vi "Scoreboard.vi"(3 "B득점":u32, 11 "A득점":u32) -> ()   [LabVIEW 2020]
panel:
  out "7SegmentB1":T1
  out "7SegmentB10":T1
  out "7SegmentB100":T1
  out "7SegmentA1":T1
  out "7SegmentA10":T1
  out "7SegmentA100":T1
  # "A득점"
  # "B득점"
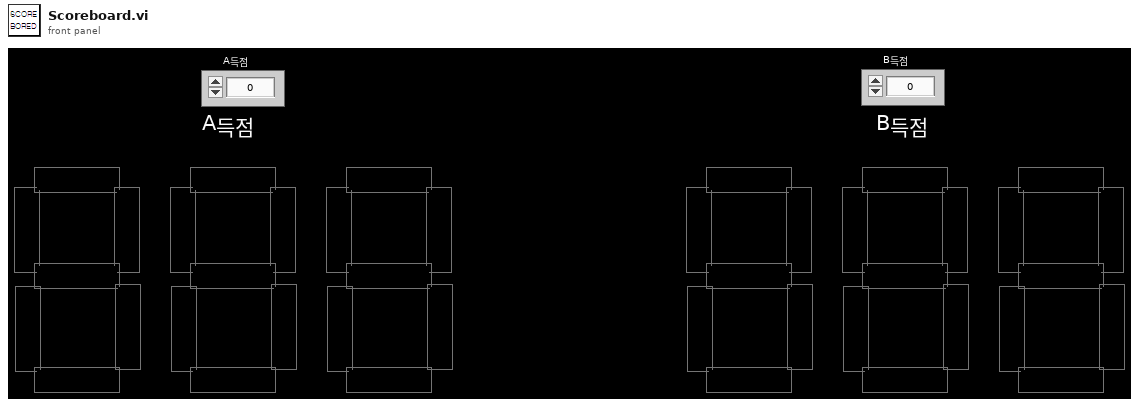
[diagram p1: front panel]
types:
  T1 = cluster{"Led 4":bool, "Led":bool, "Led 3":bool, "Led 2":bool, "Led 5":bool, "Led 6":bool, "Led 7":bool}
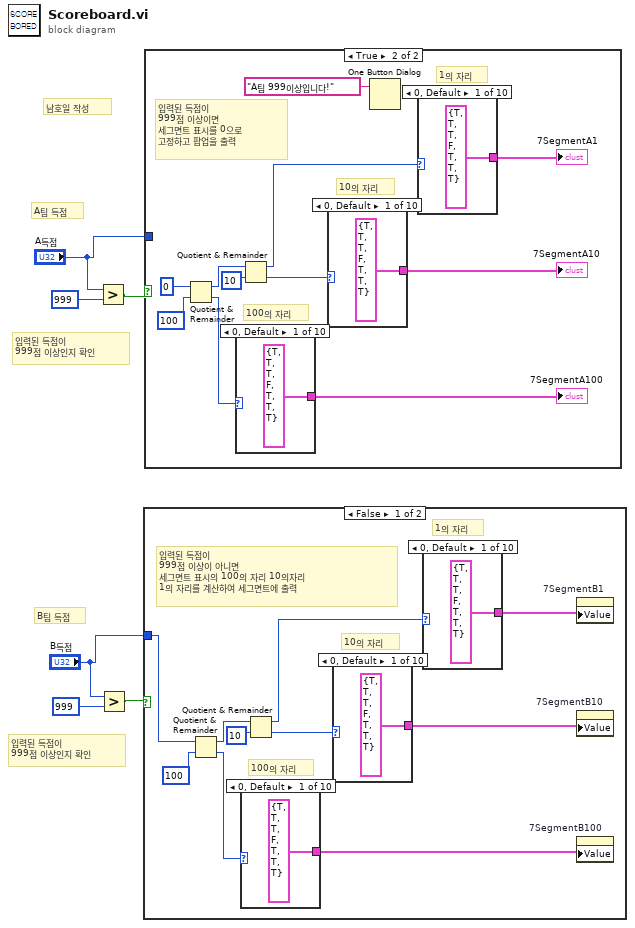
[diagram p0: block diagram]
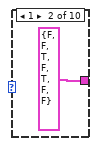
[diagram p2: hidden frame]
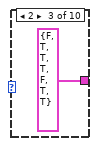
[diagram p3: hidden frame]
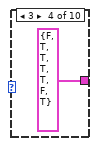
[diagram p4: hidden frame]
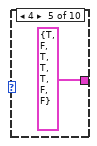
[diagram p5: hidden frame]
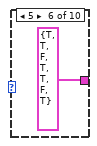
[diagram p6: hidden frame]
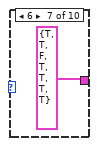
[diagram p7: hidden frame]
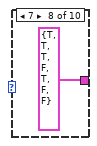
[diagram p8: hidden frame]
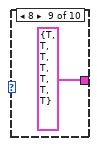
[diagram p9: hidden frame]
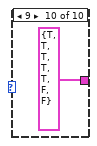
[diagram p10: hidden frame]
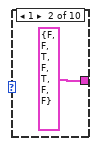
[diagram p11: hidden frame]
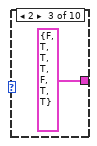
[diagram p12: hidden frame]
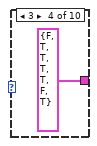
[diagram p13: hidden frame]
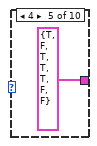
[diagram p14: hidden frame]
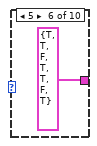
[diagram p15: hidden frame]
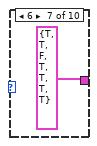
[diagram p16: hidden frame]
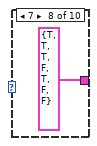
[diagram p17: hidden frame]
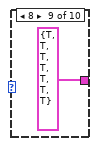
[diagram p18: hidden frame]
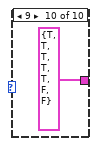
[diagram p19: hidden frame]
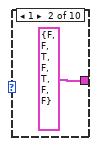
[diagram p20: hidden frame]
diagram:
  # "입력된 득점이 \n999점 이상인지 확인"
  # "입력된 득점이 \n999점 이상인지 확인"
  # "남호일 작성"
  # "B팀 득점"
  # "A팀 득점"
  n1 = Greater?(x="A득점", y=u32 999) -> (0:w2:bool)
  n2 = Greater?(x="B득점", y=u32 999) -> (0:w1:bool)
  n3 = case shown="False" w1 {
    tunnel: "B득점" -> [w7 _]
    frame False {
      # "입력된 득점이 \n999점 이상이 아니면 \n세그면트 표시의 100의 자리 10의자리 \n1의 자리를 계산하여 세그면트에 출력"
      # "1의 자리"
      # "10의 자리"
      # "100의 자리"
      n4 = Quotient & Remainder(x=w7, y=u32 100) -> (x-y*floor(x/y)=w15:u32, floor(x/y)=w14:u32)
      n5 = case shown="0, Default" w14 {
        tunnel: [T1 {"Led 4"=TRUE, "Led"=TRUE, "Led 3"=TRUE, "Led 2"=FALSE, "Led 5"=TRUE, "Led 6"=TRUE, "Led 7"=TRUE} ("7Segment10min") T1 {"Led 4"=FALSE, "Led"=FALSE, "Led 3"=TRUE, "Led 2"=FALSE, "Led 5"=TRUE, "Led 6"=FALSE, "Led 7"=FALSE} ("7Segment10min") T1 {"Led 4"=FALSE, "Led"=TRUE, "Led 3"=TRUE, "Led 2"=TRUE, "Led 5"=FALSE, "Led 6"=TRUE, "Led 7"=TRUE} ("7Segment10min") T1 {"Led 4"=FALSE, "Led"=TRUE, "Led 3"=TRUE, "Led 2"=TRUE, "Led 5"=TRUE, "Led 6"=FALSE, "Led 7"=TRUE} ("7Segment10min") T1 {"Led 4"=TRUE, "Led"=FALSE, "Led 3"=TRUE, "Led 2"=TRUE, "Led 5"=TRUE, "Led 6"=FALSE, "Led 7"=FALSE} ("7Segment10min") T1 {"Led 4"=TRUE, "Led"=TRUE, "Led 3"=FALSE, "Led 2"=TRUE, "Led 5"=TRUE, "Led 6"=FALSE, "Led 7"=TRUE} ("7Segment10min") T1 {"Led 4"=TRUE, "Led"=TRUE, "Led 3"=FALSE, "Led 2"=TRUE, "Led 5"=TRUE, "Led 6"=TRUE, "Led 7"=TRUE} ("7Segment10min") T1 {"Led 4"=TRUE, "Led"=TRUE, "Led 3"=TRUE, "Led 2"=FALSE, "Led 5"=TRUE, "Led 6"=FALSE, "Led 7"=FALSE} ("7Segment10min") T1 {"Led 4"=TRUE, "Led"=TRUE, "Led 3"=TRUE, "Led 2"=TRUE, "Led 5"=TRUE, "Led 6"=TRUE, "Led 7"=TRUE} ("7Segment10min") T1 {"Led 4"=TRUE, "Led"=TRUE, "Led 3"=TRUE, "Led 2"=TRUE, "Led 5"=TRUE, "Led 6"=FALSE, "Led 7"=FALSE} ("7Segment10min")] -> w10
        frame 0, Default {
        }
        frame 1 {
        }
        frame 2 {
        }
        frame 3 {
        }
        frame 4 {
        }
        frame 5 {
        }
        frame 6 {
        }
        frame 7 {
        }
        frame 8 {
        }
        frame 9 {
        }
      }
      n6 = Quotient & Remainder(x=w15, y=u32 10) -> (x-y*floor(x/y)=w11:u32, floor(x/y)=w12:u32)
      n7 = case shown="0, Default" w12 {
        tunnel: [T1 {"Led 4"=TRUE, "Led"=TRUE, "Led 3"=TRUE, "Led 2"=FALSE, "Led 5"=TRUE, "Led 6"=TRUE, "Led 7"=TRUE} ("7Segment10min") T1 {"Led 4"=FALSE, "Led"=FALSE, "Led 3"=TRUE, "Led 2"=FALSE, "Led 5"=TRUE, "Led 6"=FALSE, "Led 7"=FALSE} ("7Segment10min") T1 {"Led 4"=FALSE, "Led"=TRUE, "Led 3"=TRUE, "Led 2"=TRUE, "Led 5"=FALSE, "Led 6"=TRUE, "Led 7"=TRUE} ("7Segment10min") T1 {"Led 4"=FALSE, "Led"=TRUE, "Led 3"=TRUE, "Led 2"=TRUE, "Led 5"=TRUE, "Led 6"=FALSE, "Led 7"=TRUE} ("7Segment10min") T1 {"Led 4"=TRUE, "Led"=FALSE, "Led 3"=TRUE, "Led 2"=TRUE, "Led 5"=TRUE, "Led 6"=FALSE, "Led 7"=FALSE} ("7Segment10min") T1 {"Led 4"=TRUE, "Led"=TRUE, "Led 3"=FALSE, "Led 2"=TRUE, "Led 5"=TRUE, "Led 6"=FALSE, "Led 7"=TRUE} ("7Segment10min") T1 {"Led 4"=TRUE, "Led"=TRUE, "Led 3"=FALSE, "Led 2"=TRUE, "Led 5"=TRUE, "Led 6"=TRUE, "Led 7"=TRUE} ("7Segment10min") T1 {"Led 4"=TRUE, "Led"=TRUE, "Led 3"=TRUE, "Led 2"=FALSE, "Led 5"=TRUE, "Led 6"=FALSE, "Led 7"=FALSE} ("7Segment10min") T1 {"Led 4"=TRUE, "Led"=TRUE, "Led 3"=TRUE, "Led 2"=TRUE, "Led 5"=TRUE, "Led 6"=TRUE, "Led 7"=TRUE} ("7Segment10min") T1 {"Led 4"=TRUE, "Led"=TRUE, "Led 3"=TRUE, "Led 2"=TRUE, "Led 5"=TRUE, "Led 6"=FALSE, "Led 7"=FALSE} ("7Segment10min")] -> w9
        frame 0, Default {
        }
        frame 1 {
        }
        frame 2 {
        }
        frame 3 {
        }
        frame 4 {
        }
        frame 5 {
        }
        frame 6 {
        }
        frame 7 {
        }
        frame 8 {
        }
        frame 9 {
        }
      }
      n8 = case shown="0, Default" w11 {
        tunnel: [T1 {"Led 4"=TRUE, "Led"=TRUE, "Led 3"=TRUE, "Led 2"=FALSE, "Led 5"=TRUE, "Led 6"=TRUE, "Led 7"=TRUE} ("7Segment10min") T1 {"Led 4"=FALSE, "Led"=FALSE, "Led 3"=TRUE, "Led 2"=FALSE, "Led 5"=TRUE, "Led 6"=FALSE, "Led 7"=FALSE} ("7Segment10min") T1 {"Led 4"=FALSE, "Led"=TRUE, "Led 3"=TRUE, "Led 2"=TRUE, "Led 5"=FALSE, "Led 6"=TRUE, "Led 7"=TRUE} ("7Segment10min") T1 {"Led 4"=FALSE, "Led"=TRUE, "Led 3"=TRUE, "Led 2"=TRUE, "Led 5"=TRUE, "Led 6"=FALSE, "Led 7"=TRUE} ("7Segment10min") T1 {"Led 4"=TRUE, "Led"=FALSE, "Led 3"=TRUE, "Led 2"=TRUE, "Led 5"=TRUE, "Led 6"=FALSE, "Led 7"=FALSE} ("7Segment10min") T1 {"Led 4"=TRUE, "Led"=TRUE, "Led 3"=FALSE, "Led 2"=TRUE, "Led 5"=TRUE, "Led 6"=FALSE, "Led 7"=TRUE} ("7Segment10min") T1 {"Led 4"=TRUE, "Led"=TRUE, "Led 3"=FALSE, "Led 2"=TRUE, "Led 5"=TRUE, "Led 6"=TRUE, "Led 7"=TRUE} ("7Segment10min") T1 {"Led 4"=TRUE, "Led"=TRUE, "Led 3"=TRUE, "Led 2"=FALSE, "Led 5"=TRUE, "Led 6"=FALSE, "Led 7"=FALSE} ("7Segment10min") T1 {"Led 4"=TRUE, "Led"=TRUE, "Led 3"=TRUE, "Led 2"=TRUE, "Led 5"=TRUE, "Led 6"=TRUE, "Led 7"=TRUE} ("7Segment10min") T1 {"Led 4"=TRUE, "Led"=TRUE, "Led 3"=TRUE, "Led 2"=TRUE, "Led 5"=TRUE, "Led 6"=FALSE, "Led 7"=FALSE} ("7Segment10min")] -> w8
        frame 0, Default {
        }
        frame 1 {
        }
        frame 2 {
        }
        frame 3 {
        }
        frame 4 {
        }
        frame 5 {
        }
        frame 6 {
        }
        frame 7 {
        }
        frame 8 {
        }
        frame 9 {
        }
      }
      n9 = property on="7SegmentB1" class="Clust (strict)"("Value"=w8) -> ()  [unwired: 2 in, 2 out]
      n10 = property on="7SegmentB10" class="Clust (strict)"("Value"=w9) -> ()  [unwired: 2 in, 2 out]
      n11 = property on="7SegmentB100" class="Clust (strict)"("Value"=w10) -> ()  [unwired: 2 in, 2 out]
    }
    frame True {
      # "입력된 득점이 \n999점 이상이면 \n세그면트 표시를 0으로 고정하고 팝업을 출력"
      # "1의 자리"
      # "10의 자리"
      # "100의 자리"
      n12 = Quotient & Remainder(x=u32 0, y=u32 100) -> (x-y*floor(x/y)=w56:u32, floor(x/y)=w55:u32)
      n13 = case shown="0, Default" w55 {
        tunnel: [T1 {"Led 4"=TRUE, "Led"=TRUE, "Led 3"=TRUE, "Led 2"=FALSE, "Led 5"=TRUE, "Led 6"=TRUE, "Led 7"=TRUE} ("7Segment10min") T1 {"Led 4"=FALSE, "Led"=FALSE, "Led 3"=TRUE, "Led 2"=FALSE, "Led 5"=TRUE, "Led 6"=FALSE, "Led 7"=FALSE} ("7Segment10min") T1 {"Led 4"=FALSE, "Led"=TRUE, "Led 3"=TRUE, "Led 2"=TRUE, "Led 5"=FALSE, "Led 6"=TRUE, "Led 7"=TRUE} ("7Segment10min") T1 {"Led 4"=FALSE, "Led"=TRUE, "Led 3"=TRUE, "Led 2"=TRUE, "Led 5"=TRUE, "Led 6"=FALSE, "Led 7"=TRUE} ("7Segment10min") T1 {"Led 4"=TRUE, "Led"=FALSE, "Led 3"=TRUE, "Led 2"=TRUE, "Led 5"=TRUE, "Led 6"=FALSE, "Led 7"=FALSE} ("7Segment10min") T1 {"Led 4"=TRUE, "Led"=TRUE, "Led 3"=FALSE, "Led 2"=TRUE, "Led 5"=TRUE, "Led 6"=FALSE, "Led 7"=TRUE} ("7Segment10min") T1 {"Led 4"=TRUE, "Led"=TRUE, "Led 3"=FALSE, "Led 2"=TRUE, "Led 5"=TRUE, "Led 6"=TRUE, "Led 7"=TRUE} ("7Segment10min") T1 {"Led 4"=TRUE, "Led"=TRUE, "Led 3"=TRUE, "Led 2"=FALSE, "Led 5"=TRUE, "Led 6"=FALSE, "Led 7"=FALSE} ("7Segment10min") T1 {"Led 4"=TRUE, "Led"=TRUE, "Led 3"=TRUE, "Led 2"=TRUE, "Led 5"=TRUE, "Led 6"=TRUE, "Led 7"=TRUE} ("7Segment10min") T1 {"Led 4"=TRUE, "Led"=TRUE, "Led 3"=TRUE, "Led 2"=TRUE, "Led 5"=TRUE, "Led 6"=FALSE, "Led 7"=FALSE} ("7Segment10min")] -> w51
        frame 0, Default {
        }
        frame 1 {
        }
        frame 2 {
        }
        frame 3 {
        }
        frame 4 {
        }
        frame 5 {
        }
        frame 6 {
        }
        frame 7 {
        }
        frame 8 {
        }
        frame 9 {
        }
      }
      "7SegmentB100" <- w51
      n14 = Quotient & Remainder(x=w56, y=u32 10) -> (x-y*floor(x/y)=w52:u32, floor(x/y)=w53:u32)
      n15 = case shown="0, Default" w53 {
        tunnel: [T1 {"Led 4"=TRUE, "Led"=TRUE, "Led 3"=TRUE, "Led 2"=FALSE, "Led 5"=TRUE, "Led 6"=TRUE, "Led 7"=TRUE} ("7Segment10min") T1 {"Led 4"=FALSE, "Led"=FALSE, "Led 3"=TRUE, "Led 2"=FALSE, "Led 5"=TRUE, "Led 6"=FALSE, "Led 7"=FALSE} ("7Segment10min") T1 {"Led 4"=FALSE, "Led"=TRUE, "Led 3"=TRUE, "Led 2"=TRUE, "Led 5"=FALSE, "Led 6"=TRUE, "Led 7"=TRUE} ("7Segment10min") T1 {"Led 4"=FALSE, "Led"=TRUE, "Led 3"=TRUE, "Led 2"=TRUE, "Led 5"=TRUE, "Led 6"=FALSE, "Led 7"=TRUE} ("7Segment10min") T1 {"Led 4"=TRUE, "Led"=FALSE, "Led 3"=TRUE, "Led 2"=TRUE, "Led 5"=TRUE, "Led 6"=FALSE, "Led 7"=FALSE} ("7Segment10min") T1 {"Led 4"=TRUE, "Led"=TRUE, "Led 3"=FALSE, "Led 2"=TRUE, "Led 5"=TRUE, "Led 6"=FALSE, "Led 7"=TRUE} ("7Segment10min") T1 {"Led 4"=TRUE, "Led"=TRUE, "Led 3"=FALSE, "Led 2"=TRUE, "Led 5"=TRUE, "Led 6"=TRUE, "Led 7"=TRUE} ("7Segment10min") T1 {"Led 4"=TRUE, "Led"=TRUE, "Led 3"=TRUE, "Led 2"=FALSE, "Led 5"=TRUE, "Led 6"=FALSE, "Led 7"=FALSE} ("7Segment10min") T1 {"Led 4"=TRUE, "Led"=TRUE, "Led 3"=TRUE, "Led 2"=TRUE, "Led 5"=TRUE, "Led 6"=TRUE, "Led 7"=TRUE} ("7Segment10min") T1 {"Led 4"=TRUE, "Led"=TRUE, "Led 3"=TRUE, "Led 2"=TRUE, "Led 5"=TRUE, "Led 6"=FALSE, "Led 7"=FALSE} ("7Segment10min")] -> w49
        frame 0, Default {
        }
        frame 1 {
        }
        frame 2 {
        }
        frame 3 {
        }
        frame 4 {
        }
        frame 5 {
        }
        frame 6 {
        }
        frame 7 {
        }
        frame 8 {
        }
        frame 9 {
        }
      }
      "7SegmentB10" <- w49
      n16 = One Button Dialog(message="B팀 999이상입니다!") -> ()  [unwired: 1 in, 1 out]
      n17 = case shown="0, Default" w52 {
        tunnel: [T1 {"Led 4"=TRUE, "Led"=TRUE, "Led 3"=TRUE, "Led 2"=FALSE, "Led 5"=TRUE, "Led 6"=TRUE, "Led 7"=TRUE} ("7Segment10min") T1 {"Led 4"=FALSE, "Led"=FALSE, "Led 3"=TRUE, "Led 2"=FALSE, "Led 5"=TRUE, "Led 6"=FALSE, "Led 7"=FALSE} ("7Segment10min") T1 {"Led 4"=FALSE, "Led"=TRUE, "Led 3"=TRUE, "Led 2"=TRUE, "Led 5"=FALSE, "Led 6"=TRUE, "Led 7"=TRUE} ("7Segment10min") T1 {"Led 4"=FALSE, "Led"=TRUE, "Led 3"=TRUE, "Led 2"=TRUE, "Led 5"=TRUE, "Led 6"=FALSE, "Led 7"=TRUE} ("7Segment10min") T1 {"Led 4"=TRUE, "Led"=FALSE, "Led 3"=TRUE, "Led 2"=TRUE, "Led 5"=TRUE, "Led 6"=FALSE, "Led 7"=FALSE} ("7Segment10min") T1 {"Led 4"=TRUE, "Led"=TRUE, "Led 3"=FALSE, "Led 2"=TRUE, "Led 5"=TRUE, "Led 6"=FALSE, "Led 7"=TRUE} ("7Segment10min") T1 {"Led 4"=TRUE, "Led"=TRUE, "Led 3"=FALSE, "Led 2"=TRUE, "Led 5"=TRUE, "Led 6"=TRUE, "Led 7"=TRUE} ("7Segment10min") T1 {"Led 4"=TRUE, "Led"=TRUE, "Led 3"=TRUE, "Led 2"=FALSE, "Led 5"=TRUE, "Led 6"=FALSE, "Led 7"=FALSE} ("7Segment10min") T1 {"Led 4"=TRUE, "Led"=TRUE, "Led 3"=TRUE, "Led 2"=TRUE, "Led 5"=TRUE, "Led 6"=TRUE, "Led 7"=TRUE} ("7Segment10min") T1 {"Led 4"=TRUE, "Led"=TRUE, "Led 3"=TRUE, "Led 2"=TRUE, "Led 5"=TRUE, "Led 6"=FALSE, "Led 7"=FALSE} ("7Segment10min")] -> w50
        frame 0, Default {
        }
        frame 1 {
        }
        frame 2 {
        }
        frame 3 {
        }
        frame 4 {
        }
        frame 5 {
        }
        frame 6 {
        }
        frame 7 {
        }
        frame 8 {
        }
        frame 9 {
        }
      }
      "7SegmentB1" <- w50
    }
  }
  n18 = case shown="True" w2 {
    tunnel: "A득점" -> [w88 _]
    frame False {
      # "입력된 득점이 \n999점 이상이 아니면 \n세그면트 표시의 100의 자리 10의자리 \n1의 자리를 계산하여 세그면트에 출력"
      # "1의 자리"
      # "10의 자리"
      # "100의 자리"
      n19 = Quotient & Remainder(x=w88, y=u32 100) -> (x-y*floor(x/y)=w97:u32, floor(x/y)=w96:u32)
      n20 = case shown="0, Default" w96 {
        tunnel: [T1 {"Led 4"=TRUE, "Led"=TRUE, "Led 3"=TRUE, "Led 2"=FALSE, "Led 5"=TRUE, "Led 6"=TRUE, "Led 7"=TRUE} ("7Segment10min") T1 {"Led 4"=FALSE, "Led"=FALSE, "Led 3"=TRUE, "Led 2"=FALSE, "Led 5"=TRUE, "Led 6"=FALSE, "Led 7"=FALSE} ("7Segment10min") T1 {"Led 4"=FALSE, "Led"=TRUE, "Led 3"=TRUE, "Led 2"=TRUE, "Led 5"=FALSE, "Led 6"=TRUE, "Led 7"=TRUE} ("7Segment10min") T1 {"Led 4"=FALSE, "Led"=TRUE, "Led 3"=TRUE, "Led 2"=TRUE, "Led 5"=TRUE, "Led 6"=FALSE, "Led 7"=TRUE} ("7Segment10min") T1 {"Led 4"=TRUE, "Led"=FALSE, "Led 3"=TRUE, "Led 2"=TRUE, "Led 5"=TRUE, "Led 6"=FALSE, "Led 7"=FALSE} ("7Segment10min") T1 {"Led 4"=TRUE, "Led"=TRUE, "Led 3"=FALSE, "Led 2"=TRUE, "Led 5"=TRUE, "Led 6"=FALSE, "Led 7"=TRUE} ("7Segment10min") T1 {"Led 4"=TRUE, "Led"=TRUE, "Led 3"=FALSE, "Led 2"=TRUE, "Led 5"=TRUE, "Led 6"=TRUE, "Led 7"=TRUE} ("7Segment10min") T1 {"Led 4"=TRUE, "Led"=TRUE, "Led 3"=TRUE, "Led 2"=FALSE, "Led 5"=TRUE, "Led 6"=FALSE, "Led 7"=FALSE} ("7Segment10min") T1 {"Led 4"=TRUE, "Led"=TRUE, "Led 3"=TRUE, "Led 2"=TRUE, "Led 5"=TRUE, "Led 6"=TRUE, "Led 7"=TRUE} ("7Segment10min") T1 {"Led 4"=TRUE, "Led"=TRUE, "Led 3"=TRUE, "Led 2"=TRUE, "Led 5"=TRUE, "Led 6"=FALSE, "Led 7"=FALSE} ("7Segment10min")] -> w91
        frame 0, Default {
        }
        frame 1 {
        }
        frame 2 {
        }
        frame 3 {
        }
        frame 4 {
        }
        frame 5 {
        }
        frame 6 {
        }
        frame 7 {
        }
        frame 8 {
        }
        frame 9 {
        }
      }
      n21 = Quotient & Remainder(x=w97, y=u32 10) -> (x-y*floor(x/y)=w94:u32, floor(x/y)=w95:u32)
      n22 = case shown="0, Default" w95 {
        tunnel: [T1 {"Led 4"=TRUE, "Led"=TRUE, "Led 3"=TRUE, "Led 2"=FALSE, "Led 5"=TRUE, "Led 6"=TRUE, "Led 7"=TRUE} ("7Segment10min") T1 {"Led 4"=FALSE, "Led"=FALSE, "Led 3"=TRUE, "Led 2"=FALSE, "Led 5"=TRUE, "Led 6"=FALSE, "Led 7"=FALSE} ("7Segment10min") T1 {"Led 4"=FALSE, "Led"=TRUE, "Led 3"=TRUE, "Led 2"=TRUE, "Led 5"=FALSE, "Led 6"=TRUE, "Led 7"=TRUE} ("7Segment10min") T1 {"Led 4"=FALSE, "Led"=TRUE, "Led 3"=TRUE, "Led 2"=TRUE, "Led 5"=TRUE, "Led 6"=FALSE, "Led 7"=TRUE} ("7Segment10min") T1 {"Led 4"=TRUE, "Led"=FALSE, "Led 3"=TRUE, "Led 2"=TRUE, "Led 5"=TRUE, "Led 6"=FALSE, "Led 7"=FALSE} ("7Segment10min") T1 {"Led 4"=TRUE, "Led"=TRUE, "Led 3"=FALSE, "Led 2"=TRUE, "Led 5"=TRUE, "Led 6"=FALSE, "Led 7"=TRUE} ("7Segment10min") T1 {"Led 4"=TRUE, "Led"=TRUE, "Led 3"=FALSE, "Led 2"=TRUE, "Led 5"=TRUE, "Led 6"=TRUE, "Led 7"=TRUE} ("7Segment10min") T1 {"Led 4"=TRUE, "Led"=TRUE, "Led 3"=TRUE, "Led 2"=FALSE, "Led 5"=TRUE, "Led 6"=FALSE, "Led 7"=FALSE} ("7Segment10min") T1 {"Led 4"=TRUE, "Led"=TRUE, "Led 3"=TRUE, "Led 2"=TRUE, "Led 5"=TRUE, "Led 6"=TRUE, "Led 7"=TRUE} ("7Segment10min") T1 {"Led 4"=TRUE, "Led"=TRUE, "Led 3"=TRUE, "Led 2"=TRUE, "Led 5"=TRUE, "Led 6"=FALSE, "Led 7"=FALSE} ("7Segment10min")] -> w90
        frame 0, Default {
        }
        frame 1 {
        }
        frame 2 {
        }
        frame 3 {
        }
        frame 4 {
        }
        frame 5 {
        }
        frame 6 {
        }
        frame 7 {
        }
        frame 8 {
        }
        frame 9 {
        }
      }
      n23 = case shown="0, Default" w94 {
        tunnel: [T1 {"Led 4"=TRUE, "Led"=TRUE, "Led 3"=TRUE, "Led 2"=FALSE, "Led 5"=TRUE, "Led 6"=TRUE, "Led 7"=TRUE} ("7Segment10min") T1 {"Led 4"=FALSE, "Led"=FALSE, "Led 3"=TRUE, "Led 2"=FALSE, "Led 5"=TRUE, "Led 6"=FALSE, "Led 7"=FALSE} ("7Segment10min") T1 {"Led 4"=FALSE, "Led"=TRUE, "Led 3"=TRUE, "Led 2"=TRUE, "Led 5"=FALSE, "Led 6"=TRUE, "Led 7"=TRUE} ("7Segment10min") T1 {"Led 4"=FALSE, "Led"=TRUE, "Led 3"=TRUE, "Led 2"=TRUE, "Led 5"=TRUE, "Led 6"=FALSE, "Led 7"=TRUE} ("7Segment10min") T1 {"Led 4"=TRUE, "Led"=FALSE, "Led 3"=TRUE, "Led 2"=TRUE, "Led 5"=TRUE, "Led 6"=FALSE, "Led 7"=FALSE} ("7Segment10min") T1 {"Led 4"=TRUE, "Led"=TRUE, "Led 3"=FALSE, "Led 2"=TRUE, "Led 5"=TRUE, "Led 6"=FALSE, "Led 7"=TRUE} ("7Segment10min") T1 {"Led 4"=TRUE, "Led"=TRUE, "Led 3"=FALSE, "Led 2"=TRUE, "Led 5"=TRUE, "Led 6"=TRUE, "Led 7"=TRUE} ("7Segment10min") T1 {"Led 4"=TRUE, "Led"=TRUE, "Led 3"=TRUE, "Led 2"=FALSE, "Led 5"=TRUE, "Led 6"=FALSE, "Led 7"=FALSE} ("7Segment10min") T1 {"Led 4"=TRUE, "Led"=TRUE, "Led 3"=TRUE, "Led 2"=TRUE, "Led 5"=TRUE, "Led 6"=TRUE, "Led 7"=TRUE} ("7Segment10min") T1 {"Led 4"=TRUE, "Led"=TRUE, "Led 3"=TRUE, "Led 2"=TRUE, "Led 5"=TRUE, "Led 6"=FALSE, "Led 7"=FALSE} ("7Segment10min")] -> w89
        frame 0, Default {
        }
        frame 1 {
        }
        frame 2 {
        }
        frame 3 {
        }
        frame 4 {
        }
        frame 5 {
        }
        frame 6 {
        }
        frame 7 {
        }
        frame 8 {
        }
        frame 9 {
        }
      }
      n24 = property on="7SegmentA1" class="Clust (strict)"("Value"=w89) -> ()  [unwired: 2 in, 2 out]
      n25 = property on="7SegmentA10" class="Clust (strict)"("Value"=w90) -> ()  [unwired: 2 in, 2 out]
      n26 = property on="7SegmentA100" class="Clust (strict)"("Value"=w91) -> ()  [unwired: 2 in, 2 out]
    }
    frame True {
      # "입력된 득점이 \n999점 이상이면 \n세그면트 표시를 0으로 고정하고 팝업을 출력"
      # "1의 자리"
      # "10의 자리"
      # "100의 자리"
      n27 = Quotient & Remainder(x=u32 0, y=u32 100) -> (x-y*floor(x/y)=w137:u32, floor(x/y)=w136:u32)
      n28 = case shown="0, Default" w136 {
        tunnel: [T1 {"Led 4"=TRUE, "Led"=TRUE, "Led 3"=TRUE, "Led 2"=FALSE, "Led 5"=TRUE, "Led 6"=TRUE, "Led 7"=TRUE} ("7Segment10min") T1 {"Led 4"=FALSE, "Led"=FALSE, "Led 3"=TRUE, "Led 2"=FALSE, "Led 5"=TRUE, "Led 6"=FALSE, "Led 7"=FALSE} ("7Segment10min") T1 {"Led 4"=FALSE, "Led"=TRUE, "Led 3"=TRUE, "Led 2"=TRUE, "Led 5"=FALSE, "Led 6"=TRUE, "Led 7"=TRUE} ("7Segment10min") T1 {"Led 4"=FALSE, "Led"=TRUE, "Led 3"=TRUE, "Led 2"=TRUE, "Led 5"=TRUE, "Led 6"=FALSE, "Led 7"=TRUE} ("7Segment10min") T1 {"Led 4"=TRUE, "Led"=FALSE, "Led 3"=TRUE, "Led 2"=TRUE, "Led 5"=TRUE, "Led 6"=FALSE, "Led 7"=FALSE} ("7Segment10min") T1 {"Led 4"=TRUE, "Led"=TRUE, "Led 3"=FALSE, "Led 2"=TRUE, "Led 5"=TRUE, "Led 6"=FALSE, "Led 7"=TRUE} ("7Segment10min") T1 {"Led 4"=TRUE, "Led"=TRUE, "Led 3"=FALSE, "Led 2"=TRUE, "Led 5"=TRUE, "Led 6"=TRUE, "Led 7"=TRUE} ("7Segment10min") T1 {"Led 4"=TRUE, "Led"=TRUE, "Led 3"=TRUE, "Led 2"=FALSE, "Led 5"=TRUE, "Led 6"=FALSE, "Led 7"=FALSE} ("7Segment10min") T1 {"Led 4"=TRUE, "Led"=TRUE, "Led 3"=TRUE, "Led 2"=TRUE, "Led 5"=TRUE, "Led 6"=TRUE, "Led 7"=TRUE} ("7Segment10min") T1 {"Led 4"=TRUE, "Led"=TRUE, "Led 3"=TRUE, "Led 2"=TRUE, "Led 5"=TRUE, "Led 6"=FALSE, "Led 7"=FALSE} ("7Segment10min")] -> w135
        frame 0, Default {
        }
        frame 1 {
        }
        frame 2 {
        }
        frame 3 {
        }
        frame 4 {
        }
        frame 5 {
        }
        frame 6 {
        }
        frame 7 {
        }
        frame 8 {
        }
        frame 9 {
        }
      }
      "7SegmentA100" <- w135
      n29 = Quotient & Remainder(x=w137, y=u32 10) -> (x-y*floor(x/y)=w131:u32, floor(x/y)=w133:u32)
      n30 = case shown="0, Default" w133 {
        tunnel: [T1 {"Led 4"=TRUE, "Led"=TRUE, "Led 3"=TRUE, "Led 2"=FALSE, "Led 5"=TRUE, "Led 6"=TRUE, "Led 7"=TRUE} ("7Segment10min") T1 {"Led 4"=FALSE, "Led"=FALSE, "Led 3"=TRUE, "Led 2"=FALSE, "Led 5"=TRUE, "Led 6"=FALSE, "Led 7"=FALSE} ("7Segment10min") T1 {"Led 4"=FALSE, "Led"=TRUE, "Led 3"=TRUE, "Led 2"=TRUE, "Led 5"=FALSE, "Led 6"=TRUE, "Led 7"=TRUE} ("7Segment10min") T1 {"Led 4"=FALSE, "Led"=TRUE, "Led 3"=TRUE, "Led 2"=TRUE, "Led 5"=TRUE, "Led 6"=FALSE, "Led 7"=TRUE} ("7Segment10min") T1 {"Led 4"=TRUE, "Led"=FALSE, "Led 3"=TRUE, "Led 2"=TRUE, "Led 5"=TRUE, "Led 6"=FALSE, "Led 7"=FALSE} ("7Segment10min") T1 {"Led 4"=TRUE, "Led"=TRUE, "Led 3"=FALSE, "Led 2"=TRUE, "Led 5"=TRUE, "Led 6"=FALSE, "Led 7"=TRUE} ("7Segment10min") T1 {"Led 4"=TRUE, "Led"=TRUE, "Led 3"=FALSE, "Led 2"=TRUE, "Led 5"=TRUE, "Led 6"=TRUE, "Led 7"=TRUE} ("7Segment10min") T1 {"Led 4"=TRUE, "Led"=TRUE, "Led 3"=TRUE, "Led 2"=FALSE, "Led 5"=TRUE, "Led 6"=FALSE, "Led 7"=FALSE} ("7Segment10min") T1 {"Led 4"=TRUE, "Led"=TRUE, "Led 3"=TRUE, "Led 2"=TRUE, "Led 5"=TRUE, "Led 6"=TRUE, "Led 7"=TRUE} ("7Segment10min") T1 {"Led 4"=TRUE, "Led"=TRUE, "Led 3"=TRUE, "Led 2"=TRUE, "Led 5"=TRUE, "Led 6"=FALSE, "Led 7"=FALSE} ("7Segment10min")] -> w132
        frame 0, Default {
        }
        frame 1 {
        }
        frame 2 {
        }
        frame 3 {
        }
        frame 4 {
        }
        frame 5 {
        }
        frame 6 {
        }
        frame 7 {
        }
        frame 8 {
        }
        frame 9 {
        }
      }
      "7SegmentA10" <- w132
      n31 = One Button Dialog(message="A팀 999이상입니다!") -> ()  [unwired: 1 in, 1 out]
      n32 = case shown="0, Default" w131 {
        tunnel: [T1 {"Led 4"=TRUE, "Led"=TRUE, "Led 3"=TRUE, "Led 2"=FALSE, "Led 5"=TRUE, "Led 6"=TRUE, "Led 7"=TRUE} ("7Segment10min") T1 {"Led 4"=FALSE, "Led"=FALSE, "Led 3"=TRUE, "Led 2"=FALSE, "Led 5"=TRUE, "Led 6"=FALSE, "Led 7"=FALSE} ("7Segment10min") T1 {"Led 4"=FALSE, "Led"=TRUE, "Led 3"=TRUE, "Led 2"=TRUE, "Led 5"=FALSE, "Led 6"=TRUE, "Led 7"=TRUE} ("7Segment10min") T1 {"Led 4"=FALSE, "Led"=TRUE, "Led 3"=TRUE, "Led 2"=TRUE, "Led 5"=TRUE, "Led 6"=FALSE, "Led 7"=TRUE} ("7Segment10min") T1 {"Led 4"=TRUE, "Led"=FALSE, "Led 3"=TRUE, "Led 2"=TRUE, "Led 5"=TRUE, "Led 6"=FALSE, "Led 7"=FALSE} ("7Segment10min") T1 {"Led 4"=TRUE, "Led"=TRUE, "Led 3"=FALSE, "Led 2"=TRUE, "Led 5"=TRUE, "Led 6"=FALSE, "Led 7"=TRUE} ("7Segment10min") T1 {"Led 4"=TRUE, "Led"=TRUE, "Led 3"=FALSE, "Led 2"=TRUE, "Led 5"=TRUE, "Led 6"=TRUE, "Led 7"=TRUE} ("7Segment10min") T1 {"Led 4"=TRUE, "Led"=TRUE, "Led 3"=TRUE, "Led 2"=FALSE, "Led 5"=TRUE, "Led 6"=FALSE, "Led 7"=FALSE} ("7Segment10min") T1 {"Led 4"=TRUE, "Led"=TRUE, "Led 3"=TRUE, "Led 2"=TRUE, "Led 5"=TRUE, "Led 6"=TRUE, "Led 7"=TRUE} ("7Segment10min") T1 {"Led 4"=TRUE, "Led"=TRUE, "Led 3"=TRUE, "Led 2"=TRUE, "Led 5"=TRUE, "Led 6"=FALSE, "Led 7"=FALSE} ("7Segment10min")] -> w130
        frame 0, Default {
        }
        frame 1 {
        }
        frame 2 {
        }
        frame 3 {
        }
        frame 4 {
        }
        frame 5 {
        }
        frame 6 {
        }
        frame 7 {
        }
        frame 8 {
        }
        frame 9 {
        }
      }
      "7SegmentA1" <- w130
    }
  }
